vi "Configure Noise Characteristics.vi"(6 "Noise Removal (F: Disable)":bool, 7 "Enable Random Noise (F: Disable)":bool, 8 "error in (no error)":errorcluster, 9 "Report Method (0: Spectral)":i32(ring) items=["Spectral", "Tail Fit"], 10 "Random Noise Method (0: Spectral)":i32(ring) items=["Spectral", "Both"], 11 "VISA resource name":refnum<visa-resource-name>) -> (0 "error out":errorcluster, 3 "VISA resource name out":refnum<visa-resource-name>)   [LabVIEW 2020, in "Agilent 90000 Series.lvlib"]
doc: "Configure random noise settings of noise measurement.\n\n<B>Note:</B>\nThis control is only available when the EZJIT Complete software is installed."
uses:
  Agilent 90000 Series.lvlib
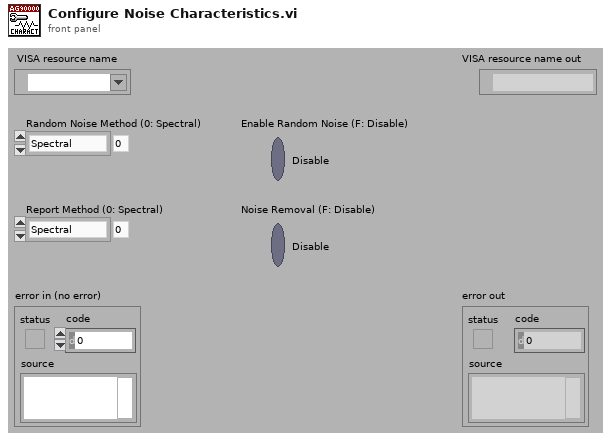
[diagram p1: front panel]
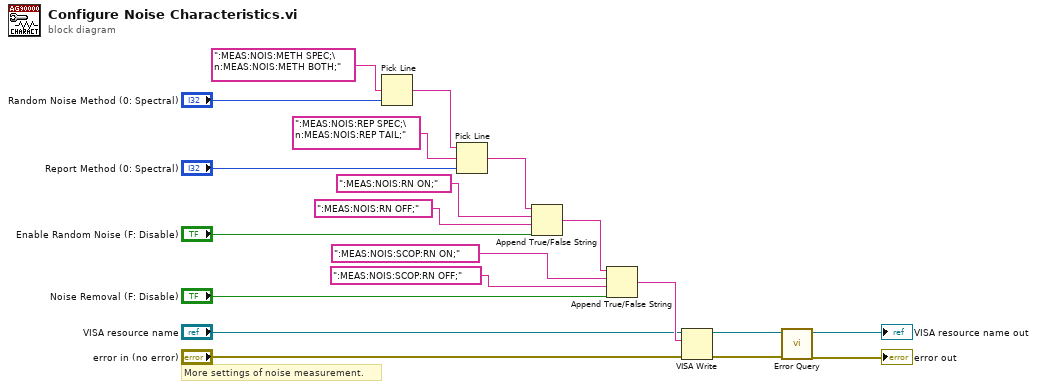
[diagram p0: block diagram]
diagram:
  # "More settings of noise measurement."
  n1 = Pick Line(multi-line string=":MEAS:NOIS:METH SPEC;\n:MEAS:NOIS:METH BOTH;", line index="Random Noise Method (0: Spectral)") -> (output string=w16:string)  [unwired: 1 out]
  n2 = Pick Line(string ("")=w16, multi-line string=":MEAS:NOIS:REP SPEC;\n:MEAS:NOIS:REP TAIL;", line index="Report Method (0: Spectral)") -> (output string=w15:string)
  n3 = Append True/False String(1:"Enable Random Noise (F: Disable)", 2:":MEAS:NOIS:RN OFF;", 3:":MEAS:NOIS:RN ON;", 4:w15) -> (0:w11:string)
  n4 = Append True/False String(1:"Noise Removal (F: Disable)", 2:":MEAS:NOIS:SCOP:RN OFF;", 3:":MEAS:NOIS:SCOP:RN ON;", 4:w11) -> (0:w7:string)
  n5 = VISA Write(VISA resource name="VISA resource name", write buffer=w7, error in (no error)="error in (no error)") -> (VISA resource name out=w4:refnum<visa-resource-name>, error out=w3:errorcluster)  [unwired: 1 out]
  n6 = call "Error Query.vi"("error in (no error)"=w3, "VISA resource name"=w4) -> ("error out"=→"error out":errorcluster, "VISA resource name out"=→"VISA resource name out":refnum<visa-resource-name>)  [unwired: 8 out]
